vi "Read DB Connection String.vi"(8 "error in (no error)":errorcluster, 11 "CS++Factory in":refnum<class "CS++Factory.lvclass">) -> (0 "error out":errorcluster, 2 "DB Connection String":string, 3 "CS++Factory out":refnum<class "CS++Factory.lvclass">)   [LabVIEW 2013, in "CS++BaseClasses.lvlib" / "CS++Factory.lvclass"]
doc: "Read DB Connection String."
uses:
  CS++Factory.lvclass
  CS++Factory.lvclass/CS++Factory.ctl
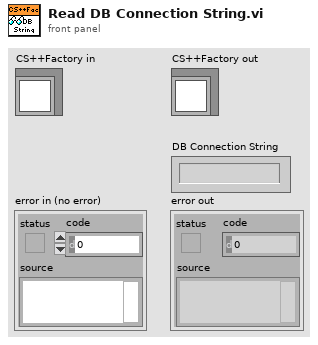
[diagram p1: front panel]
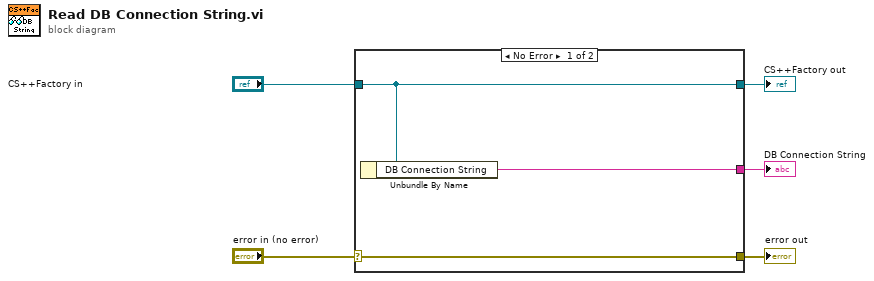
[diagram p0: block diagram]
diagram:
  n1 = case shown="No Error" "error in (no error)" {
    selector: "error in (no error)" -> [w8 w9]
    tunnel: [w8 w9] -> w4
    tunnel: [w7 w10] -> w2
    tunnel: "CS++Factory in" -> [w7 w10]
    tunnel: [w6 _] -> w1
    frame No Error {
      n2 = Unbundle By Name(w7) -> ("DB Connection String"=w6:string)
    }
    frame Error {
    }
  }
  "error out" <- w4
  "CS++Factory out" <- w2
  "DB Connection String" <- w1
